vi "ArduinoLDC500GUI.vi"() -> ()   [LabVIEW 2017]
doc: "Use this template to build a user interface event handler design pattern. Use this pattern for dialog boxes and other user interfaces. You also can create and execute user-defined events that the VI can handle the same way as user interface events."
uses:
  <vilib>/Utility/config.llb/Read Key (String).vi
  <vilib>/Instr/_visa.llb/VISA Configure Serial Port (Instr).vi
  <vilib>/Utility/config.llb/Write Key (String).vi
  <vilib>/Utility/config.llb/NI_LVConfig.lvlib
panel:
  in  "HIGH":bool
  in  "LOW":bool
  out "time":string
  out "LaserOn":bool
  out "SerialNumber":string
  in  "SetCurrent [mA]":i32(slide) min=0 max=250 step=2 scale=0.0..260.0
  out "635nm [mW]":dbl(slide) scale=0.1..140.0 scale format="%#1_1p"
  in  "ComPort":refnum<visa-resource-name>
  in  "Shutter_On_Off":bool
  in  "stop":bool
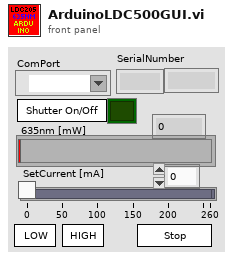
[diagram p1: front panel]
types:
  T1 = typedef "NI_LVConfig.lvlib/Config Data RefNum.ctl" = refnum<k1>
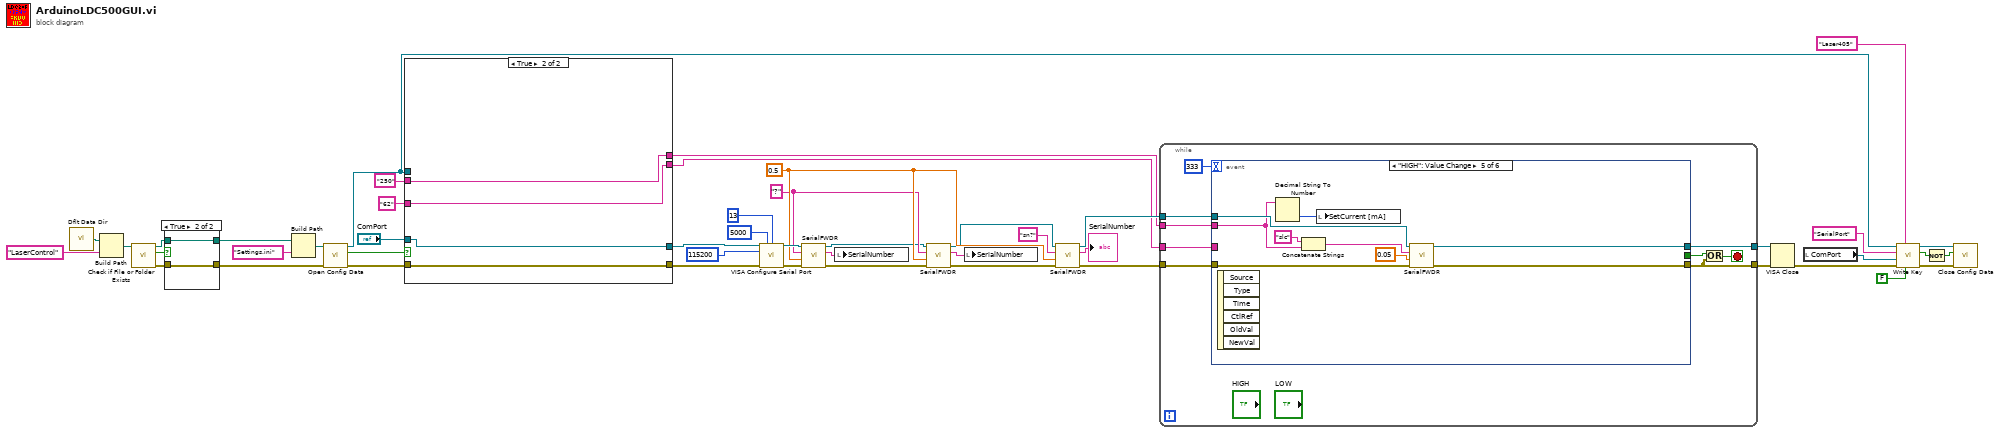
[diagram p0: block diagram]
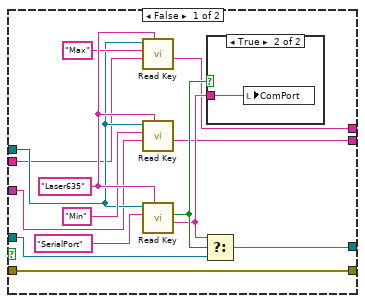
[diagram p2: hidden frame]
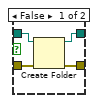
[diagram p4: hidden frame]
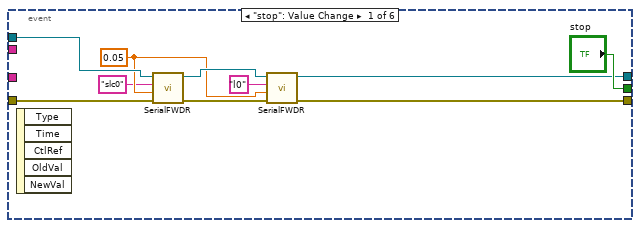
[diagram p5: hidden frame]
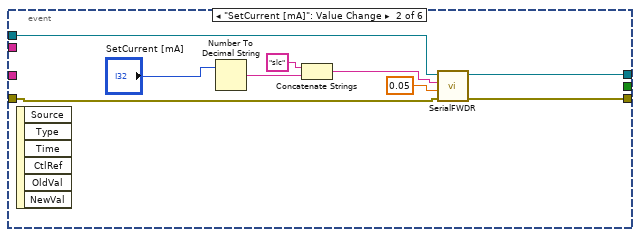
[diagram p6: hidden frame]
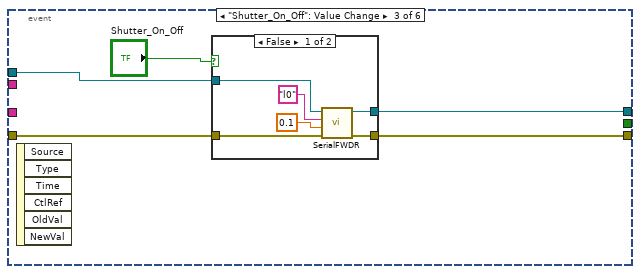
[diagram p7: hidden frame]
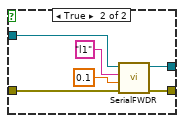
[diagram p8: hidden frame]
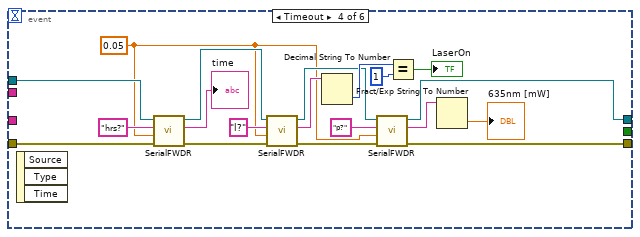
[diagram p9: hidden frame]
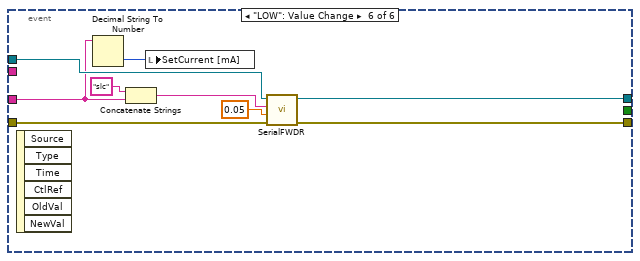
[diagram p10: hidden frame]
diagram:
  w12 = "?" ("CommandString")
  w13 = 0.5 ("Delay Time (s)")
  n1 = call <vilib>:"Dflt Data Dir.vi"() -> ("App:Default Data Directory"=w42:path)
  n2 = Build Path(base path=w42, name or relative path="LaserControl") -> (appended path=w39:path)
  n3 = call <vilib>:"Check if File or Folder Exists.vi"("path"=w39) -> ("error out"=w36:errorcluster, "file or folder exists?"=w38:bool, "dup path"=w37:path)  [unwired: 8 in]
  n4 = case shown="True" w38 {
    tunnel: [w51 w54] -> w34
    tunnel: w37 -> [w52 w54]
    tunnel: w36 -> [w50 w53]
    tunnel: [w49 w53] -> w35
    frame False {
      n5 = Create Folder(path (use dialog)=w52, error in=w50) -> (created path=w51:path, error out=w49:errorcluster)  [unwired: 1 in, 1 out]
    }
    frame True {
    }
  }
  n6 = Build Path(base path=w34, name or relative path="Settings.ini") -> (appended path=w40:path)
  n7 = call <vilib>:"Open Config Data.vi"("error in (no error)"=w35, "configuration file path"=w40) -> ("error out"=w32:errorcluster, "file created?"=w29:bool, "refnum"=w30:T1)  [unwired: 7 in]
  n8 = case shown="True" w29 {
    tunnel: "ComPort" -> [w65 w73]
    tunnel: w32 -> [w64 w72]
    tunnel: w30 -> [w59 _]
    tunnel: [w64 w72] -> w22
    tunnel: [w63 w73] -> w26
    tunnel: [w58 w71] -> w4
    tunnel: [w57 w70] -> w3
    tunnel: "62" ("default value") -> [w56 w71]
    tunnel: "250" ("default value") -> [w55 w70]
    frame False {
      w62 = "Laser635" ("section")
      n9 = call-poly <vilib>:"Read Key.vi"("section"=w62, "default value"=w55, "key"="Max", "refnum"=w59) -> ("value"=w57:string)  [unwired: 4 in, 3 out]
      n10 = call-poly <vilib>:"Read Key.vi"("section"=w62, "default value"=w56, "key"="Min", "refnum"=w59) -> ("value"=w58:string)  [unwired: 4 in, 3 out]
      n11 = call-poly <vilib>:"Read Key.vi"("section"=w62, "key"="SerialPort", "refnum"=w59) -> ("value"=w66:string, "found?"=w67:bool)  [unwired: 5 in, 2 out]
      n12 = Select(t=w66, s=w67, f=w65) -> (s? t:f=w63:string)
      n13 = case shown="True" w67 {
        tunnel: w66 -> [_ w69]
        frame False {
        }
        frame True {
          n14 = local write "ComPort"(w69) -> ()
        }
      }
    }
    frame True {
    }
  }
  n15 = call-poly "VISA Configure Serial Port"("VISA resource name"=w26, "timeout (10sec)"=u32 5000, "termination char\n(0xA = '\\n' = LF)"=u8 13 ("termination char\n(0xA = '\\n' = LF)"), "baud rate (9600)"=u32 115200, "error in (no error)"=w22) -> ("VISA resource name out"=w16:refnum<visa-resource-name>, "error out"=w15:errorcluster)  [unwired: 9 in]
  n16 = call "SerialFWDR.vi"("error in (no error)"=w15, "Delay Time (s)"=w13, "CommandString"=w12, "VISA Refnum in"=w16) -> ("error out"=w8:errorcluster, "trimmed string"=w14:string, "VISA Refnum out"=w11:refnum<visa-resource-name>)  [unwired: 5 in]
  n17 = local write "SerialNumber"(w14) -> ()
  n18 = call "SerialFWDR.vi"("error in (no error)"=w8, "Delay Time (s)"=w13, "CommandString"=w12, "VISA Refnum in"=w11) -> ("error out"=w7:errorcluster, "trimmed string"=w9:string, "VISA Refnum out"=w10:refnum<visa-resource-name>)  [unwired: 5 in]
  n19 = local write "SerialNumber"(w9) -> ()
  n20 = call "SerialFWDR.vi"("error in (no error)"=w7, "Delay Time (s)"=w13, "CommandString"="sn?", "VISA Refnum in"=w10) -> ("error out"=w6:errorcluster, "trimmed string"=→"SerialNumber":string, "VISA Refnum out"=w5:refnum<visa-resource-name>)  [unwired: 5 in]
  n21 = while {
    tunnel: w5 -> [w81]
    tunnel: w6 -> [w80]
    tunnel: [w77] -> w19
    tunnel: [w82] -> w18
    tunnel: w4 -> [w75]
    tunnel: w3 -> [w74]
    stop <- w78 stop-if-true
    n22 = event shown="[4] \"HIGH\": Value Change" {
      selector: _ -> [_ _ _ _ _ _]
      dyn-events: _ -> [_ _ _ _ _ _]
      timeout: 333 -> [_ _ _ _ _ _]
      tunnel: ["stop" _ _ _ _ _] -> w76
      tunnel: [w90 w96 w103 w119 w142 w151] -> w77
      tunnel: w80 -> [w88 w97 w104 w136 w144 w153]
      tunnel: [w91 w98 w106 w120 w143 w152] -> w82
      tunnel: w81 -> [w86 w99 w105 w137 w145 w154]
      tunnel: w75 -> [_ _ _ _ _ w148]
      tunnel: w74 -> [_ _ _ _ w138 _]
      event "stop": Value Change {
        w84 = 0.05 ("Delay Time (s)")
        n23 = event-data() -> ()  [unwired: 1 in, 5 out]
        n24 = call "SerialFWDR.vi"("error in (no error)"=w88, "Delay Time (s)"=w84, "CommandString"="slc0", "VISA Refnum in"=w86) -> ("error out"=w87:errorcluster, "VISA Refnum out"=w85:refnum<visa-resource-name>)  [unwired: 5 in, 1 out]
        n25 = call "SerialFWDR.vi"("error in (no error)"=w87, "Delay Time (s)"=w84, "CommandString"="l0", "VISA Refnum in"=w85) -> ("error out"=w90:errorcluster, "VISA Refnum out"=w91:refnum<visa-resource-name>)  [unwired: 5 in, 1 out]
      }
      event "SetCurrent [mA]": Value Change {
        n26 = event-data() -> ()  [unwired: 1 in, 6 out]
        n27 = Number To Decimal String(number="SetCurrent [mA]") -> (decimal integer string=w100:string)  [unwired: 1 in]
        n28 = Concatenate Strings("slc" ("string"), w100) -> (w95:string)
        n29 = call "SerialFWDR.vi"("error in (no error)"=w97, "Delay Time (s)"=0.05, "CommandString"=w95, "VISA Refnum in"=w99) -> ("error out"=w96:errorcluster, "VISA Refnum out"=w98:refnum<visa-resource-name>)  [unwired: 5 in, 1 out]
      }
      event "Shutter_On_Off": Value Change {
        n30 = event-data() -> ()  [unwired: 1 in, 6 out]
        n31 = case shown="False" "Shutter_On_Off" {
          tunnel: [w112 w117] -> w106
          tunnel: w105 -> [w108 w118]
          tunnel: w104 -> [w107 w116]
          tunnel: [w111 w115] -> w103
          frame False {
            n32 = call "SerialFWDR.vi"("error in (no error)"=w107, "Delay Time (s)"=0.1, "CommandString"="l0", "VISA Refnum in"=w108) -> ("error out"=w111:errorcluster, "VISA Refnum out"=w112:refnum<visa-resource-name>)  [unwired: 5 in, 1 out]
          }
          frame True {
            n33 = call "SerialFWDR.vi"("error in (no error)"=w116, "Delay Time (s)"=0.1, "CommandString"="l1", "VISA Refnum in"=w118) -> ("error out"=w115:errorcluster, "VISA Refnum out"=w117:refnum<visa-resource-name>)  [unwired: 5 in, 1 out]
          }
        }
      }
      event Timeout {
        w123 = 0.05 ("Delay Time (s)")
        n34 = event-data() -> ()  [unwired: 1 in, 3 out]
        n35 = call "SerialFWDR.vi"("error in (no error)"=w136, "Delay Time (s)"=w123, "CommandString"="hrs?", "VISA Refnum in"=w137) -> ("error out"=w132:errorcluster, "trimmed string"=→"time":string, "VISA Refnum out"=w133:refnum<visa-resource-name>)  [unwired: 5 in]
        n36 = call "SerialFWDR.vi"("error in (no error)"=w132, "Delay Time (s)"=w123, "CommandString"="l?", "VISA Refnum in"=w133) -> ("error out"=w125:errorcluster, "trimmed string"=w128:string, "VISA Refnum out"=w126:refnum<visa-resource-name>)  [unwired: 5 in]
        n37 = Decimal String To Number(string=w128) -> (number=w129:i32)  [unwired: 2 in, 1 out]
        n38 = call "SerialFWDR.vi"("error in (no error)"=w125, "Delay Time (s)"=w123, "CommandString"="p?", "VISA Refnum in"=w126) -> ("error out"=w119:errorcluster, "trimmed string"=w122:string, "VISA Refnum out"=w120:refnum<visa-resource-name>)  [unwired: 5 in]
        n39 = Equal?(x=w129, y=1) -> (x = y?=→"LaserOn":bool)
        n40 = Fract/Exp String To Number(string=w122) -> (number=→"635nm [mW]":dbl)  [unwired: 3 in, 1 out]
      }
      event "HIGH": Value Change {
        n41 = event-data() -> ()  [unwired: 1 in, 6 out]
        n42 = Decimal String To Number(string=w138) -> (number=w141:i32)  [unwired: 2 in, 1 out]
        n43 = Concatenate Strings("slc" ("string"), w138) -> (w140:string)
        n44 = local write "SetCurrent [mA]"(w141) -> ()
        n45 = call "SerialFWDR.vi"("error in (no error)"=w144, "Delay Time (s)"=0.05, "CommandString"=w140, "VISA Refnum in"=w145) -> ("error out"=w142:errorcluster, "VISA Refnum out"=w143:refnum<visa-resource-name>)  [unwired: 5 in, 1 out]
      }
      event "LOW": Value Change {
        n46 = event-data() -> ()  [unwired: 1 in, 6 out]
        n47 = Decimal String To Number(string=w148) -> (number=w147:i32)  [unwired: 2 in, 1 out]
        n48 = Concatenate Strings("slc" ("string"), w148) -> (w149:string)
        n49 = local write "SetCurrent [mA]"(w147) -> ()
        n50 = call "SerialFWDR.vi"("error in (no error)"=w153, "Delay Time (s)"=0.05, "CommandString"=w149, "VISA Refnum in"=w154) -> ("error out"=w151:errorcluster, "VISA Refnum out"=w152:refnum<visa-resource-name>)  [unwired: 5 in, 1 out]
      }
    }
    n51 = Or(x=w76, y=w77) -> (x .or. y?=w78:bool)
  }
  n52 = VISA Close(VISA resource name=w18, error in (no error)=w19) -> (error out=w17:errorcluster)
  n53 = local read "ComPort"() -> (w45:refnum<visa-resource-name>)
  n54 = call-poly <vilib>:"Write Key.vi"("write raw string? (F)"=FALSE, "section"="Laser405", "error in (no error)"=w17, "value"=w45, "key"="SerialPort", "refnum"=w30) -> ("error out"=w43:errorcluster, "found?"=w28:bool, "refnum out"=w44:T1)  [unwired: 3 in]
  n55 = Not(x=w28) -> (.not. x?=w27:bool)
  n56 = call <vilib>:"Close Config Data.vi"("error in (no error)"=w43, "write file if changed (T)"=w27, "refnum"=w44) -> ()  [unwired: 7 in, 2 out]
